vi "Wait_Case_Arg.vi"(5 "Specific Argument":string, 6 "seconds since 1Jan1904":dbl) -> (0 "Error Comments":string, 3 "Minutes To Wait":dbl format="%.1f")   [LabVIEW 2010]
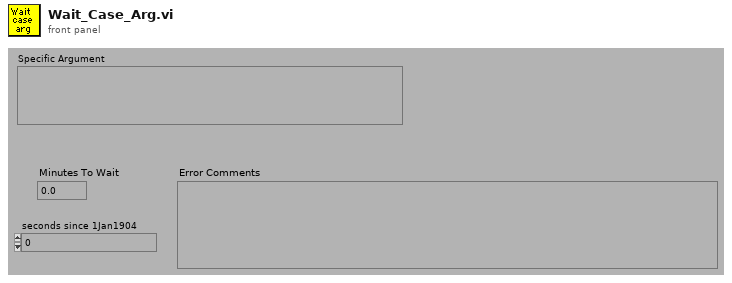
[diagram p1: front panel]
types:
  T1 = cluster{"second":i32, "minute":i32, "hour":i32, "day of month":i32, "month":i32, "year":i32, "day of week":i32, "day of year":i32, "is DST":i32}
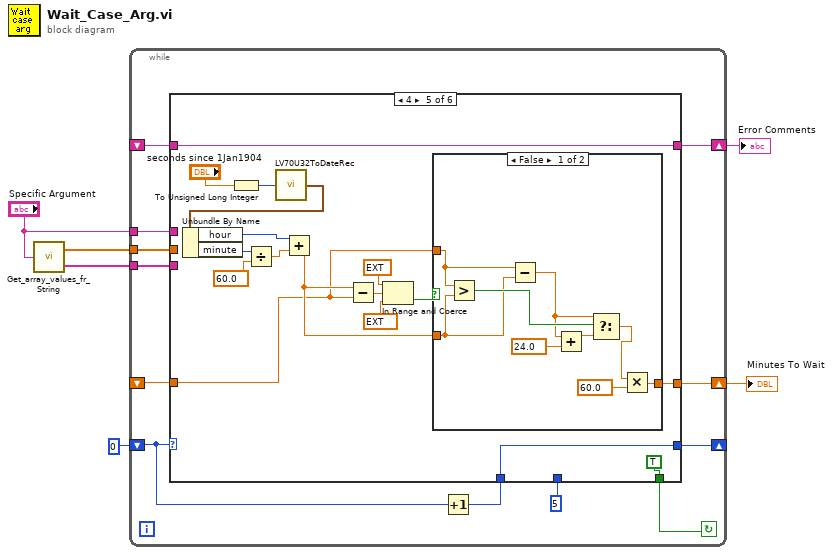
[diagram p0: block diagram]
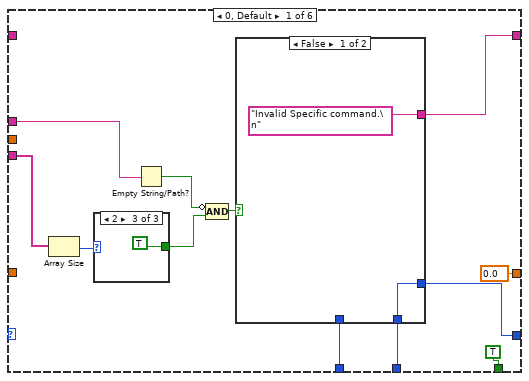
[diagram p2: hidden frame]
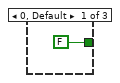
[diagram p3: hidden frame]
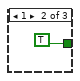
[diagram p4: hidden frame]
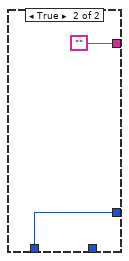
[diagram p5: hidden frame]
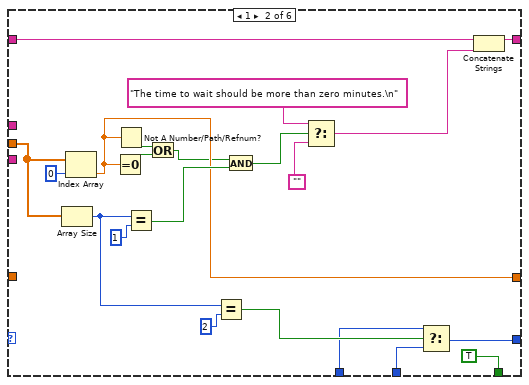
[diagram p6: hidden frame]
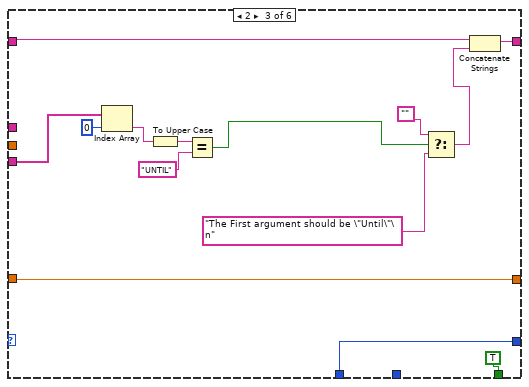
[diagram p7: hidden frame]
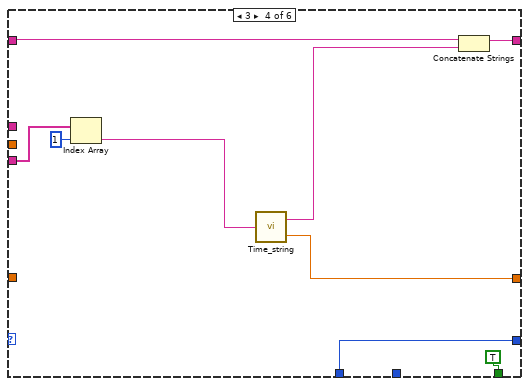
[diagram p8: hidden frame]
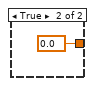
[diagram p9: hidden frame]
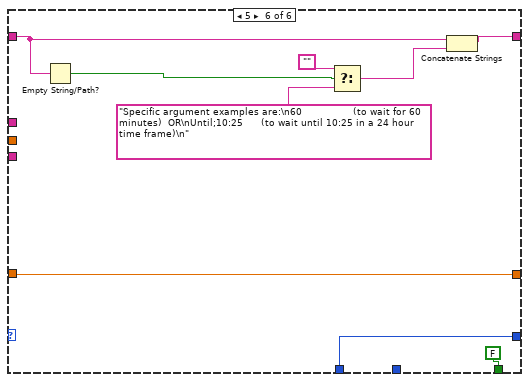
[diagram p10: hidden frame]
diagram:
  n1 = call "Get_array_values_fr_String.vi"("String Value"="Specific Argument") -> ("Numeric Array"=w3:dbl[], "String array"=w5:string[])
  n2 = while {
    tunnel: "Specific Argument" -> [w7]
    shift-left: _ -> [w8]
    shift-right: [w9] -> w2
    tunnel: w3 -> [w11]
    shift-left: _ -> [w12]
    shift-right: [w13] -> w4
    tunnel: w5 -> [w18]
    shift-left: 0 -> [w17]
    shift-right: [w15] -> _
    stop <- w14 continue-if-true
    n3 = Increment(x=w17) -> (x+1=w16:i32)
    n4 = case shown="4" w17 {
      tunnel: w18 -> [w24 _ w64 w75 _ _]
      tunnel: w16 -> [w28 w43 w69 w80 w98 w110]
      tunnel: [w29 w48 w69 w80 w98 w110] -> w15
      tunnel: [TRUE TRUE TRUE TRUE TRUE FALSE] -> w14
      tunnel: [w30 w56 w66 w77 w96 w112] -> w13
      tunnel: w12 -> [_ w57 w67 w78 w96 w114]
      tunnel: w11 -> [_ w53 _ _ _ _]
      tunnel: 5 ("t") -> [w26 w42 _ _ _ _]
      tunnel: [0.0 w41 w59 w73 w86 w111] -> w9
      tunnel: w8 -> [_ _ w59 _ w84 w111]
      tunnel: w7 -> [w23 _ _ _ _ _]
      frame 0, Default {
        n5 = Array Size(array=w24) -> (size(s)=w22:i32)
        n6 = case shown="2" w22 {
          tunnel: [FALSE TRUE TRUE] -> w20
          frame 0, Default {
          }
          frame 1 {
          }
          frame 2 {
          }
        }
        n7 = Empty String/Path?(string/path=w23) -> (empty?=w21:bool)
        n8 = Compound Arithmetic op=AND(invert w21, w20) -> (w19:bool)
        n9 = case shown="False" w19 {
          tunnel: ["Invalid Specific command.\n" ""] -> w30
          tunnel: [w34 w36] -> w29
          tunnel: w28 -> [_ w36]
          tunnel: w26 -> [w34 _]
          frame False {
          }
          frame True {
          }
        }
      }
      frame 1 {
        n10 = Array Size(array=w53) -> (size(s)=w45:i32)
        n11 = Index Array(array=w53, index=0 ("Index")) -> (element=w41:dbl)
        n12 = Equal To 0?(x=w41) -> (x = 0?=w40:bool)
        n13 = Not A Number/Path/Refnum?(number/path/refnum=w41) -> (NaN/Path/Refnum?=w39:bool)
        n14 = Equal?(x=w45, y=1) -> (x = y?=w47:bool)
        n15 = Or(x=w39, y=w40) -> (x .or. y?=w38:bool)
        n16 = Equal?(x=w45, y=2) -> (x = y?=w44:bool)
        n17 = And(x=w38, y=w47) -> (x .and. y?=w51:bool)
        n18 = Select(t="The time to wait should be more than zero minutes.\n", s=w51, f="") -> (s? t:f=w52:string)
        n19 = Select(t=w43, s=w44, f=w42) -> (s? t:f=w48:i32)
        n20 = Concatenate Strings(w57, w52) -> (w56:string)
      }
      frame 2 {
        n21 = Index Array(array=w64, index=0 ("Index")) -> (element=w63:string)
        n22 = To Upper Case(1:w63) -> (0:w62:string)
        n23 = Equal?(x=w62, y="UNTIL") -> (x = y?=w60:bool)
        n24 = Select(t="", s=w60, f="The First argument should be \"Until\"\n" ("Format String")) -> (s? t:f=w65:string)
        n25 = Concatenate Strings(w67, w65) -> (w66:string)
      }
      frame 3 {
        n26 = Index Array(array=w75, index=1 ("Index")) -> (element=w74:string)
        n27 = call "Time_string.vi"("Input String"=w74) -> ("Error String"=w76:string, "24 Hour decimal"=w73:dbl)
        n28 = Concatenate Strings(w78, w76) -> (w77:string)
      }
      frame 4 {
        n29 = To Unsigned Long Integer(number="seconds since 1Jan1904") -> (unsigned 32bit integer=w82:u32)
        n30 = call <vilib>:"LV70U32ToDateRec.vi"("Time"=w82) -> ("date time rec"=w95:T1)
        n31 = Unbundle By Name(w95) -> ("hour"=w92:i32, "minute"=w94:i32)
        n32 = Divide(x=w94, y=60.0) -> (x/y=w91:dbl)
        n33 = Add(x=w92, y=w91) -> (x+y=w85:dbl)
        n34 = Subtract(x=w85, y=w84) -> (x-y=w90:dbl)
        n35 = In Range and Coerce(upper limit=ext 4.0 ("hi"), x=w90, lower limit=ext -0.01 ("lo")) -> (In Range?=w87:bool)  [unwired: 1 out]
        n36 = case shown="False" w87 {
          tunnel: [w100 0.0] -> w86
          tunnel: w84 -> [w106 _]
          tunnel: w85 -> [w105 _]
          frame False {
            n37 = Greater?(x=w106, y=w105) -> (0:w107:bool)
            n38 = Subtract(x=w106, y=w105) -> (x-y=w102:dbl)
            n39 = Add(x=w102, y=24.0) -> (x+y=w103:dbl)
            n40 = Select(t=w102, s=w107, f=w103) -> (s? t:f=w101:dbl)
            n41 = Multiply(x=w101, y=60.0) -> (x*y=w100:dbl)
          }
          frame True {
          }
        }
      }
      frame 5 {
        n42 = Empty String/Path?(string/path=w114) -> (empty?=w117:bool)
        n43 = Select(t="", s=w117, f="Specific argument examples are:\n60                 (to wait for 60 minutes)  OR\nUntil;10:25      (to wait until 10:25 in a 24 hour time frame)\n") -> (s? t:f=w115:string)
        n44 = Concatenate Strings(w114, w115) -> (w112:string)
      }
    }
  }
  "Error Comments" <- w4
  "Minutes To Wait" <- w2
